vi "Configure Diameter.vi"(0 "VISA resource name":refnum<visa-resource-name>="COM1", 5 "Address (00)":i32 format="%02.0f", 9 "Diameter (8.66 mm)":dbl=8.66, 11 "error in (no error)":errorcluster) -> (4 "VISA resource name out":refnum<visa-resource-name>, 6 "Pump status":T1 items=["Error - Can't read status"=-1, "Stopped"=0, "Infusing"=1, "Withdrawing"=2, "Pump stalled"=3, "Stopped at infuse limit"=4, "Stopped at withdraw limit"=5, "Emergency stop"=6, "Stopped at target volume"=7], 10 "Output String":string, 15 "error out":errorcluster)   [LabVIEW 2011]
doc: "This VI sets the syringe diameter, units are mm. The inside diameter (ID) should be used for this measurement.\n\nIf you do not know your syringe diameter, refer to appendix B of the manual for nominal inside diameters of most popular syringes. For the greatest accuracy or if your syringe is not listed in appendix B, measure the inside diameter with a vernier caliper or other precision measuring tool. Record this value for future use.\n\nNote:\n(1) Rate is set to zero after this VI is run.\n\nModified from original which is Copyright 2005, National Instruments Corporation.\n\nModifications Copyright 2009, Jeff Gelles, Brandeis University"
uses:
  Pump status.ctl
panel:
  out "Command string":string
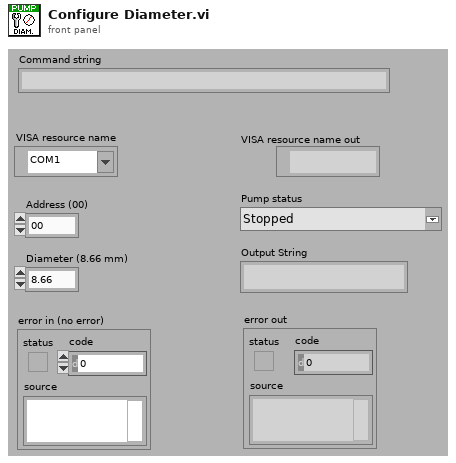
[diagram p1: front panel]
types:
  T1 = typedef "Pump status.ctl" = i8
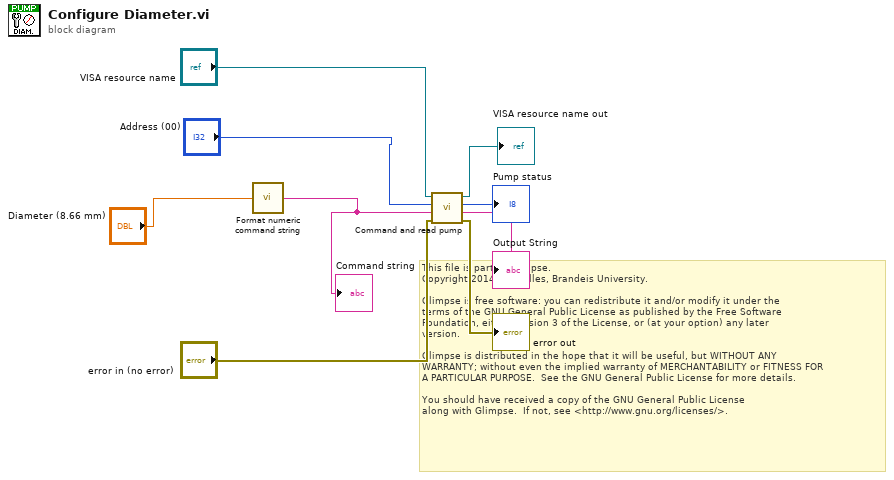
[diagram p0: block diagram]
diagram:
  # "This file is part of Glimpse. \nCopyright 2014 Jeff Gelles, Brandeis University.    \n\nGlimpse is free software: you can redistribute it and/or modify it under the \nterms of the GNU General Public License as published by the Free Software \nFoundation, either version 3 of the License, or (at your option) any later \nversion.\n\nGlimpse is distributed in the hope that it will be useful, but WITHOUT ANY \nWARRANTY; without even the implied warranty of MERCHANTABILITY or FITNESS FOR \nA PARTICULAR PURPOSE.  See the GNU General Public License for more details.\n\nYou should have received a copy of the GNU General Public License\nalong with Glimpse.  If not, see <http://www.gnu.org/licenses/>."
  n1 = call "Format numeric command string.vi"("Number"="Diameter (8.66 mm)") -> ("String"=w8:string)
  "Command string" <- w8
  n2 = call "Command and read pump.vi"("error in (no error)"="error in (no error)", "command"=w8, "Address (00)"="Address (00)", "VISA resource name"="VISA resource name") -> ("error out"=→"error out":errorcluster, "Output String"=→"Output String":string, "Pump status"=→"Pump status":T1, "VISA resource name out"=→"VISA resource name out":refnum<visa-resource-name>)
